vi "多反-头缺检测-边线检测.vi"(8 "缺损最大偏移量":dbl=0.995260663507109 format="%#_13g", 9 "Annulus":T3={"Center X"=305, "Center Y"=239, "Inner Radius"=89, "Outer Radius"=238, "Start Angle"=0.0, "End Angle"=0.0} {"End Angle" min=-90.0 max=90.0 step=1.0 format="%.2f"; "Start Angle" min=-90.0 max=90.0 step=1.0 format="%.2f"; "Center X" scale=0.0..1024.0}, 11 "IMG_IN":T4(plugin-control)) -> (0 "Defect Points":cluster{"X":dbl, "Y":dbl}[](array[cluster]), 1 "Pass Status":bool, 2 "最大值":dbl, 3 "IMG_OUT":T4(plugin-control))   [LabVIEW 2018]
doc: "This example shows a contour analysis application. The contour of the rim of the can is extracted and a circle is fitted to those points. Then the contour is compared to the fitted circle to locate defects."
uses:
  <vilib>/vision/Contour.llb/IMAQ Contour Curve Extraction.ctl
  <vilib>/vision/NI_Vision_Development_Module.lvlib
panel:
  out "error out":errorcluster
  in  "Curve Extraction":T1={"Extraction Mode"=0, "Edge Threshold"=70, "Edge Filter Size"=2, "Min Length"=50, "Search Step Size"=15, "Max Endpoint Gap"=10, "Subpixel"=TRUE} {"Extraction Mode" items=["Normal", "Uniform Regions"]; "Edge Filter Size" items=["Fine", "Normal", "Contour Tracing"]; "Max Endpoint Gap" min=0; "Search Step Size" min=1 max=255 step=1; "Min Length" min=0; "Edge Threshold" min=1 max=350 step=1}
  in  "显示边线情况":bool
  in  "Contour Equation Settings":T2={"Overlay?"=TRUE, "Color"=3381759, "Width"=1, "Maintain Width?"=TRUE}
  in  "Contour Points Settings":T2={"Overlay?"=TRUE, "Color"=6618880, "Width"=1, "Maintain Width?"=TRUE}
  in  "error in (no error)":errorcluster
  out "Distance":dbl[](graph) caption="Distance of Contour from Fitted Circle"
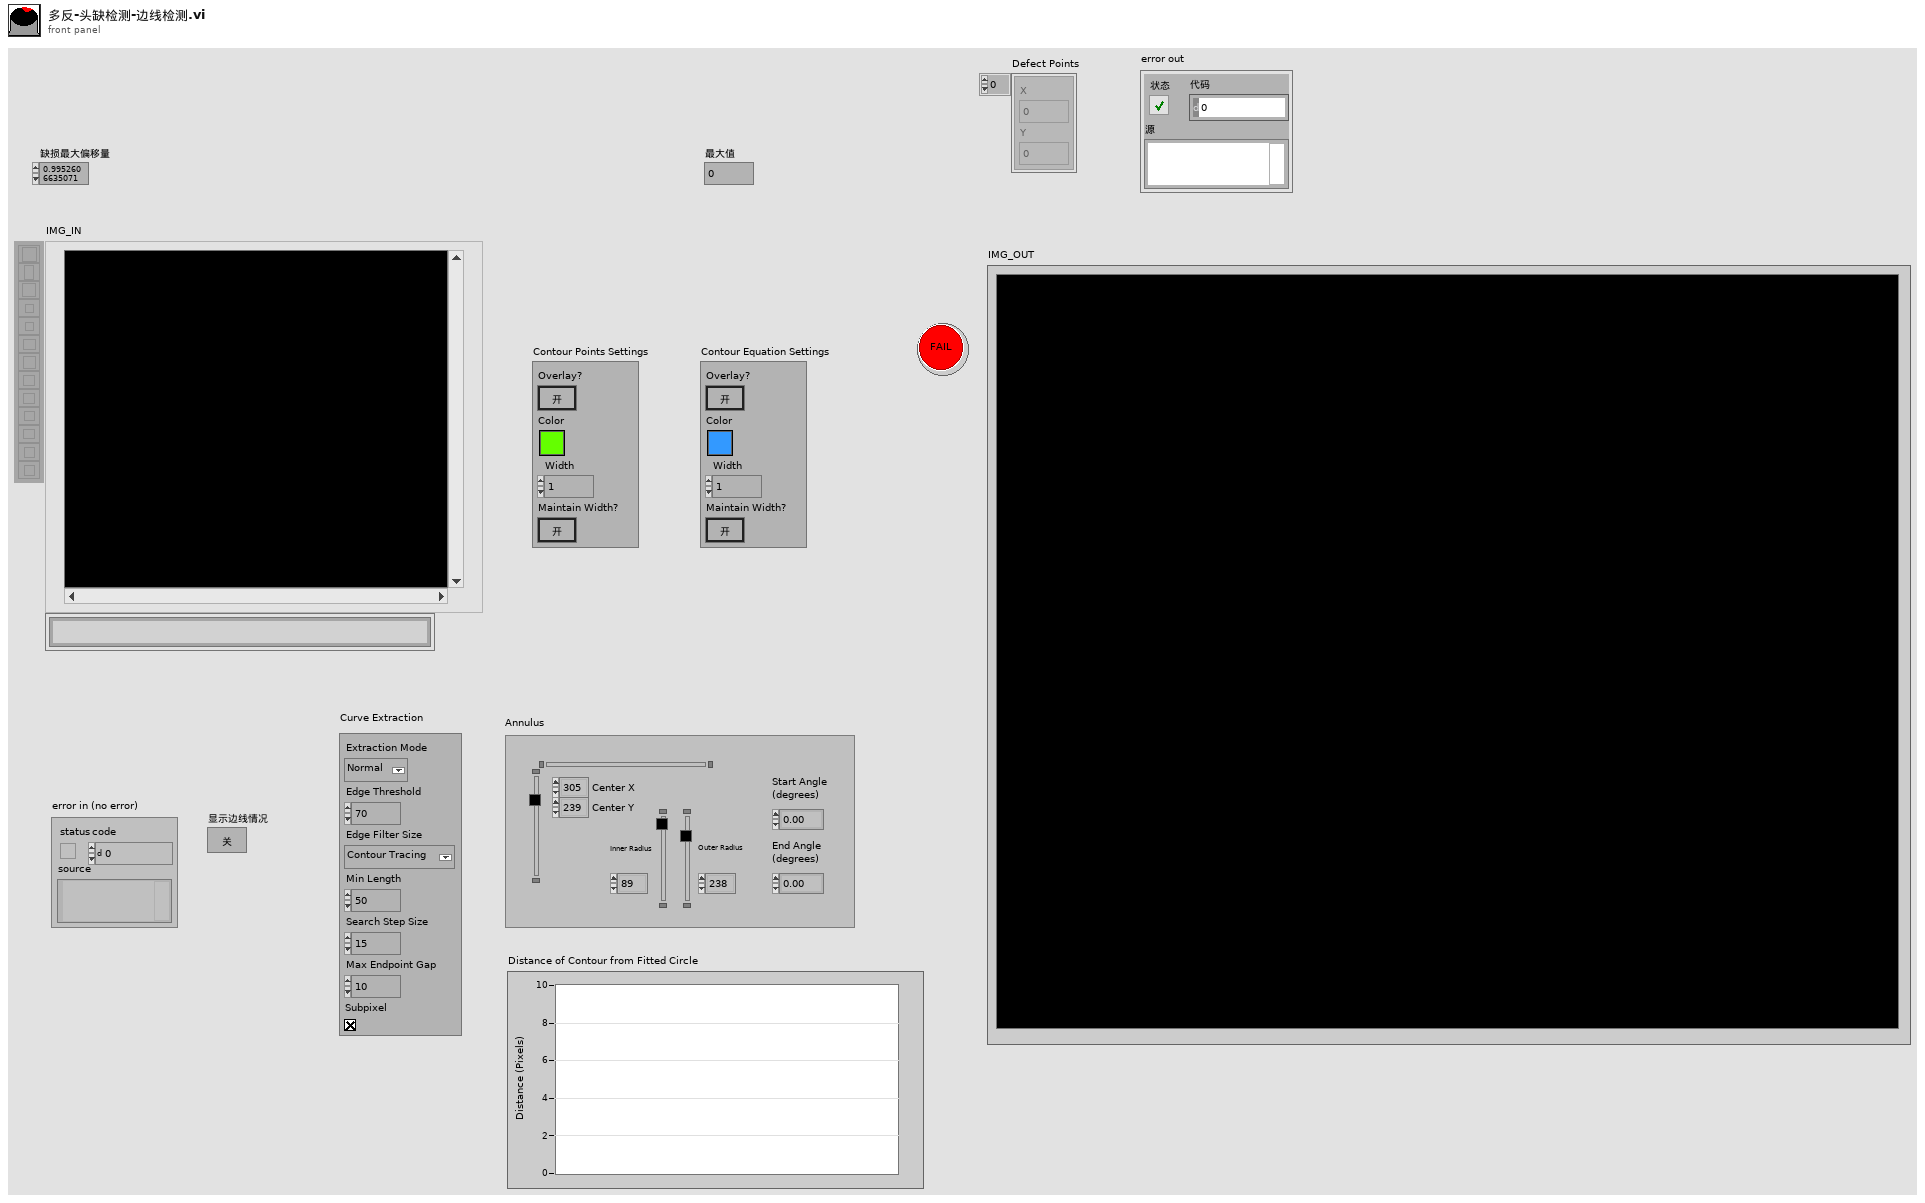
[diagram p1: front panel]
types:
  T1 = typedef "IMAQ Contour Curve Extraction.ctl" = cluster{"Extraction Mode":u32, "Edge Threshold":i32, "Edge Filter Size":u32, "Min Length":i32, "Search Step Size":i32, "Max Endpoint Gap":i32, "Subpixel":bool}
  T2 = cluster{"Overlay?":bool, "Color":u32, "Width":u32, "Maintain Width?":bool}
  T3 = typedef "IMAQ Circle" = cluster{"Center X":i32, "Center Y":i32, "Inner Radius":i32, "Outer Radius":i32, "Start Angle":dbl, "End Angle":dbl}
  T4 = typedef "IMAQ Image.ctl" = refnum<image>
  T5 = enum16{"Closest To Search Start", "Maximum Length", "Strongest Mean Gradient Change"}
  T6 = enum16{"Rect Left To Right", "Rect Right To Left", "Rect Top To Bottom", "Rect Bottom To Top", "Annulus Inner To Outer", "Annulus Outer To Inner", "Annulus Start Angle To End Angle", "Annulus End Angle To Start Angle"}
  T7 = typedef "ROI Descriptor" = cluster{"Global Rectangle":i32[], "Contours":cluster{"ID":enum32{"External", "Internal"}, "Type":u32, "Coordinates":i32[]}[]}
  T8 = cluster{"Target Point":cluster{"X":dbl, "Y":dbl}, "Template Point":cluster{"X":dbl, "Y":dbl}, "Distance":dbl}[]
  T9 = cluster{"Target Point":cluster{"X":dbl, "Y":dbl}, "Template Point":cluster{"X":dbl, "Y":dbl}, "Distance":dbl}
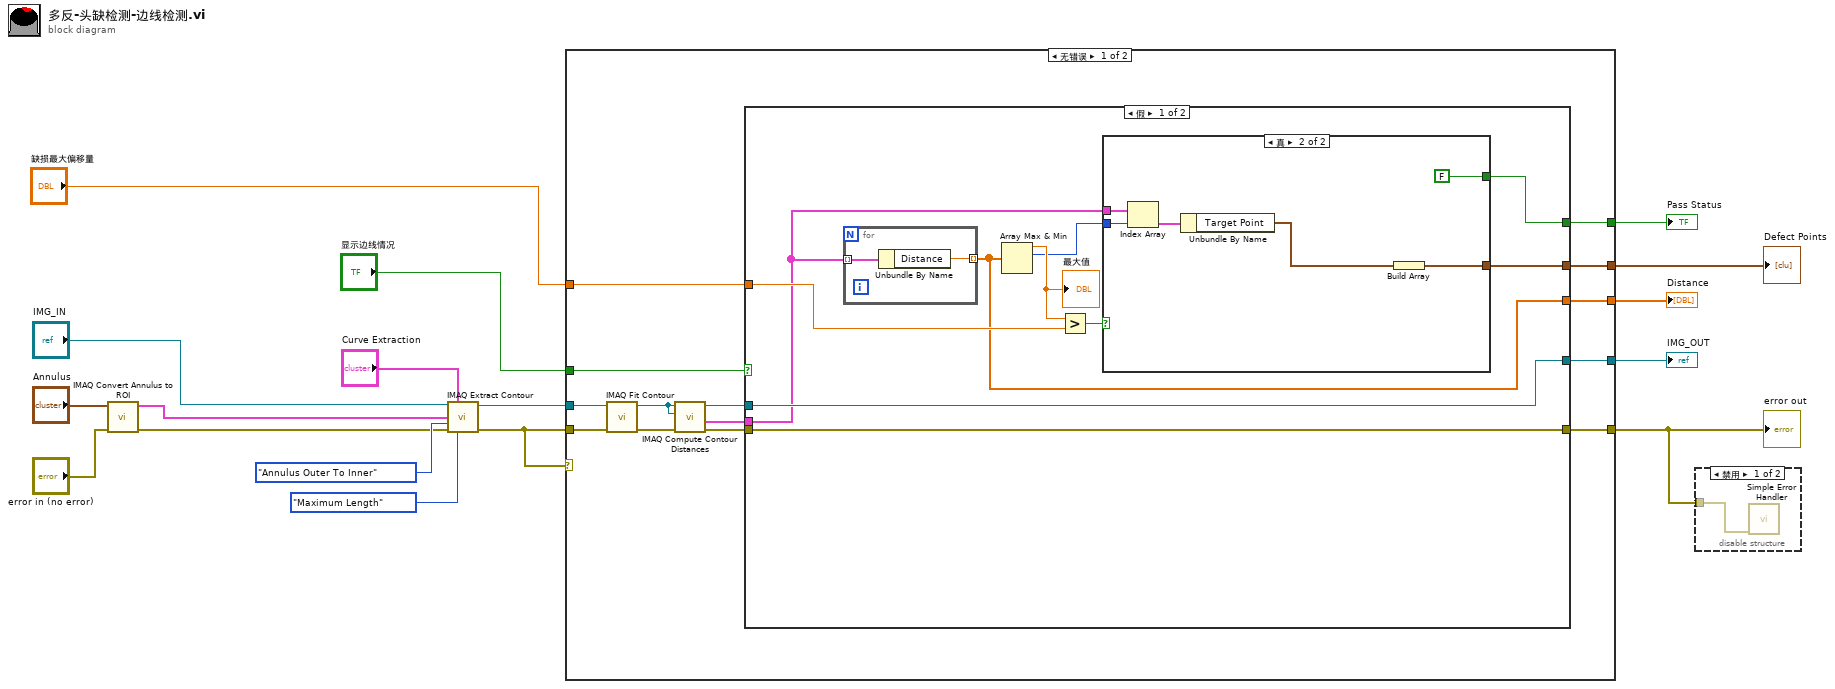
[diagram p0: block diagram]
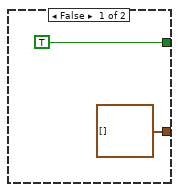
[diagram p3: hidden frame]
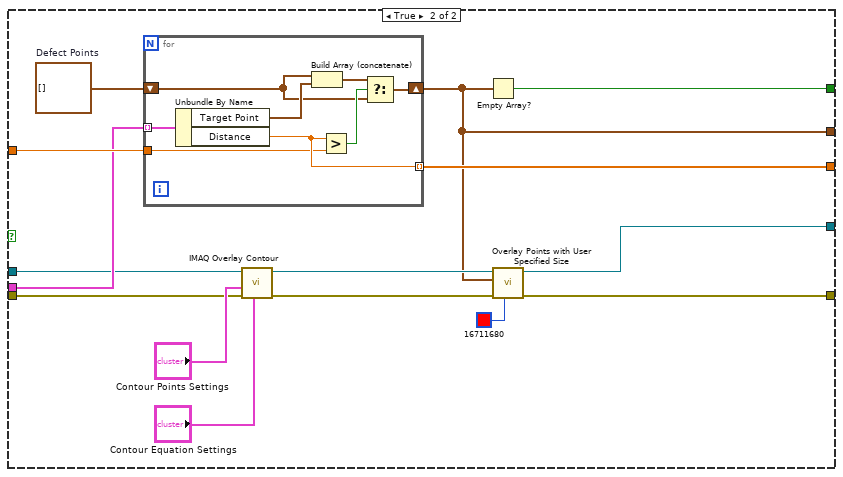
[diagram p4: hidden frame]
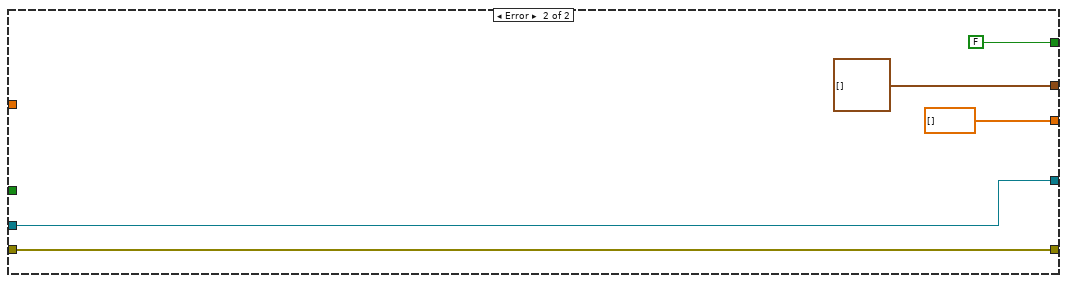
[diagram p5: hidden frame]
diagram:
  n1 = call "IMAQ Convert Annulus to ROI"("error in (no error)"="error in (no error)", "Annulus"="Annulus") -> ("error out"=w11:errorcluster, "ROI Descriptor"=w2:T7)  [unwired: 7 in]
  n2 = call "IMAQ Extract Contour"("Source Image"="IMG_IN", "Curve Extraction"="Curve Extraction", "ROI Descriptor"=w2, "Search Direction"=T6."Annulus Outer To Inner", "error in (no error)"=w11, "Contour Selection"=T5."Maximum Length") -> ("Source Image Out"=w4:T4, "error out"=w3:errorcluster)  [unwired: 2 in, 6 out]
  n3 = case shown="无错误" w3 {
    tunnel: [w31 w78] -> w17
    tunnel: w4 -> [w22 w78]
    tunnel: [w30 dbl[] []] -> w13
    tunnel: [w29 FALSE ("empty?")] -> w12
    tunnel: "缺损最大偏移量" -> [w28 _]
    tunnel: [w27 w79] -> w8
    tunnel: "显示边线情况" -> [w26 _]
    tunnel: w3 -> [w20 w79]
    tunnel: [w25 cluster{"X":dbl, "Y":dbl}[] [] ("Defect Points")] -> w6
    frame No Error {
      n4 = call-poly "IMAQ Fit Contour"("error in (no error)"=w20, "Contour Image"=w22) -> ("error out"=w23:errorcluster, "Contour Image Out"=w24:T4)  [unwired: 2 in, 6 out]
      n5 = call "IMAQ Compute Contour Distances"("error in (no error)"=w23, "Template Contour Image"=w24, "Target Contour Image"=w24) -> ("error out"=w19:errorcluster, "Distances"=w18:T8, "Target Contour Image Out (dup)"=w21:T4)  [unwired: 2 in, 4 out]
      n6 = case shown="假" w26 {
        tunnel: [w34 w66] -> w31
        tunnel: w21 -> [w34 w52]
        tunnel: w19 -> [w35 w53]
        tunnel: [w36 w60] -> w30
        tunnel: [w37 w59] -> w29
        tunnel: w28 -> [w40 w57]
        tunnel: [w35 w56] -> w27
        tunnel: [w33 w55] -> w25
        tunnel: w18 -> [w32 w54]
        frame False {
          n7 = for {
            tunnel: w32 -> [w51] mode=indexing
            tunnel: [w50] -> w36 mode=indexing
            n8 = Unbundle By Name(w51) -> ("Distance"=w50:dbl)
          }
          n9 = Array Max & Min(array=w36) -> (max value=w41:dbl, max index (indices)=w39:i32)  [unwired: 2 out]
          "最大值" <- w41
          n10 = Greater?(x=w41, y=w40) -> (0:w38:bool)
          n11 = case shown="真" w38 {
            tunnel: w32 -> [_ w49]
            tunnel: w39 -> [_ w48]
            tunnel: [TRUE FALSE] -> w37
            tunnel: [cluster{"X":dbl, "Y":dbl}[] [] w44] -> w33
            frame False {
            }
            frame True {
              n12 = Index Array(array=w49, index=w48) -> (element=w47:T9)
              n13 = Unbundle By Name(w47) -> ("Target Point"=w45:cluster{"X":dbl, "Y":dbl})
              n14 = Build Array(w45) -> (w44:cluster{"X":dbl, "Y":dbl}[])
            }
          }
        }
        frame True {
          w63 = cluster{"X":dbl, "Y":dbl}[] []  # Defect Points
          n15 = for {
            tunnel: w54 -> [w74] mode=indexing
            shift-right: [w69] -> w55
            shift-left: w63 -> [w70]
            tunnel: [w68] -> w60 mode=indexing
            tunnel: w57 -> [w67]
            n16 = Unbundle By Name(w74) -> ("Target Point"=w73:cluster{"X":dbl, "Y":dbl}, "Distance"=w68:dbl)
            n17 = Build Array (concatenate)(w70, w73) -> (w71:cluster{"X":dbl, "Y":dbl}[])
            n18 = Greater?(x=w68, y=w67) -> (0:w72:bool)
            n19 = Select(t=w71, s=w72, f=w70) -> (s? t:f=w69:cluster{"X":dbl, "Y":dbl}[])
          }
          n20 = call "IMAQ Overlay Contour"("Contour Equation Settings"="Contour Equation Settings", "error in (no error)"=w53, "Contour Points Settings"="Contour Points Settings", "Image"=w52) -> ("error out"=w58:errorcluster, "Image Out"=w62:T4)  [unwired: 2 in, 4 out]
          n21 = Empty Array?(array=w55) -> (empty?=w59:bool)
          n22 = call "Overlay Points with User Specified Size.vi"("Color"=u32 16711680, "error in"=w58, "Points"=w55, "Image In"=w62) -> ("error out"=w56:errorcluster, "Image Out"=w66:T4)  [unwired: 6 in]
        }
      }
    }
    frame Error {
    }
  }
  "IMG_OUT" <- w17
  "Distance" <- w13
  "Pass Status" <- w12
  "Defect Points" <- w6
  "error out" <- w8
  n23 = disable-structure shown="禁用" {
    disable-tunnel: w8 -> [w80 _]
    frame Disabled {
      n24 = call <vilib>:"Simple Error Handler.vi"("error in (no error)"=w80) -> ()  [unwired: 4 in, 5 out]
    }
    frame Enabled {
    }
  }
